vi "Tosca-Enqueue Dequeue Timing Test.vi"() -> ()   [LabVIEW 2015]
panel:
  out "x-y":u32
  in  "stop":bool
  out "Trials":i32
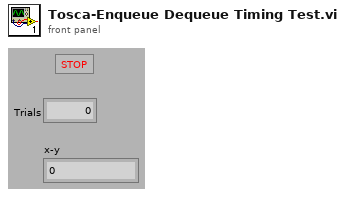
[diagram p1: front panel]
types:
  T1 = cluster{"millisecond timer value":u32, dbl[][], bool[][]}
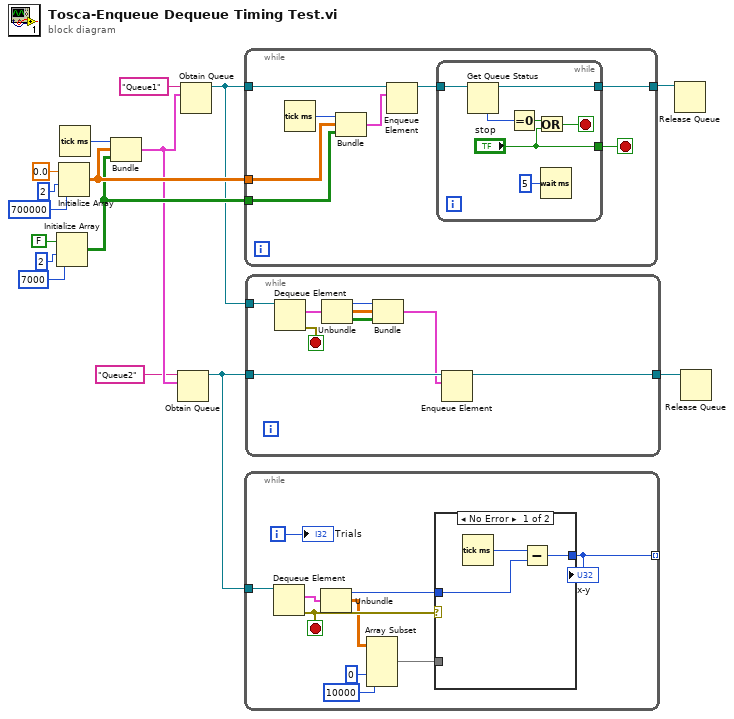
[diagram p0: block diagram]
diagram:
  n1 = Initialize Array(FALSE, 2 ("dimension size"), 7000 ("dimension size")) -> (w7:bool[][])
  n2 = Initialize Array(0.0 ("element"), 2 ("dimension size"), 700000 ("dimension size")) -> (w11:dbl[][])
  n3 = Tick Count (ms)() -> (millisecond timer value=w12:u32)
  n4 = Bundle("millisecond timer value"=w12, w11, w7) -> (w5:T1)  [unwired: 1 in]
  n5 = Obtain Queue(name (unnamed)="Queue2", element data type=w5) -> (queue out=w2:refnum<queue>)  [unwired: 3 in, 2 out]
  n6 = Obtain Queue(name (unnamed)="Queue1", element data type=w5) -> (queue out=w6:refnum<queue>)  [unwired: 3 in, 2 out]
  n7 = while {
    tunnel: w6 -> [w21]
    tunnel: [w22] -> w16
    tunnel: w11 -> [w19]
    tunnel: w7 -> [w17]
    stop <- w24 stop-if-true
    n8 = Tick Count (ms)() -> (millisecond timer value=w23:u32)
    n9 = Bundle("millisecond timer value"=w23, w19, w17) -> (w18:T1)  [unwired: 1 in]
    n10 = Enqueue Element(queue=w21, element=w18) -> (queue out=w20:refnum<queue>)  [unwired: 2 in, 2 out]
    n11 = while {
      tunnel: w20 -> [w31]
      tunnel: [w30] -> w22
      tunnel: ["stop"] -> w24
      stop <- w27 stop-if-true
      n12 = Get Queue Status(queue=w31) -> (queue out=w30:refnum<queue>, # elements in queue=w29:i32)  [unwired: 2 in, 6 out]
      n13 = Equal To 0?(x=w29) -> (x = 0?=w28:bool)
      n14 = Or(x=w28, y="stop") -> (x .or. y?=w27:bool)
      n15 = Wait (ms)(milliseconds to wait=u32 5) -> ()  [unwired: 1 out]
    }
  }
  n16 = while {
    tunnel: w2 -> [w41]
    tunnel: [w39] -> _ mode=indexing
    i -> [w40]
    stop <- w38 stop-if-true
    n17 = Dequeue Element(queue=w41) -> (element=w37:T1, error out=w38:errorcluster)  [unwired: 2 in, 2 out]
    n18 = Unbundle(w37) -> ("millisecond timer value"=w36:u32, w35:dbl[][])  [unwired: 1 out]
    n19 = Array Subset(array=w35, index (col)=0 ("index"), length (col)=10000 ("length")) -> (w32:dbl[][])  [unwired: 2 in]
    n20 = case shown="No Error" w38 {
      tunnel: [w43 _] -> w39
      tunnel: w36 -> [w42 _]
      tunnel: w32 -> [_ _]
      frame No Error {
        n21 = Tick Count (ms)() -> (millisecond timer value=w44:u32)
        n22 = Subtract(x=w44, y=w42) -> (x-y=w43:u32)
      }
      frame Error {
      }
    }
    "x-y" <- w39
    "Trials" <- w40
  }
  n23 = while {
    tunnel: w6 -> [w53]
    tunnel: w2 -> [w47]
    tunnel: [w45] -> w1
    stop <- w52 stop-if-true
    n24 = Dequeue Element(queue=w53) -> (element=w51:T1, error out=w52:errorcluster)  [unwired: 2 in, 2 out]
    n25 = Unbundle(w51) -> ("millisecond timer value"=w50:u32, w49:dbl[][], w48:bool[][])
    n26 = Bundle("millisecond timer value"=w50, w49, w48) -> (w46:T1)  [unwired: 1 in]
    n27 = Enqueue Element(queue=w47, element=w46) -> (queue out=w45:refnum<queue>)  [unwired: 2 in, 2 out]
  }
  n28 = Release Queue(queue=w16) -> ()  [unwired: 2 in, 3 out]
  n29 = Release Queue(queue=w1) -> ()  [unwired: 2 in, 3 out]
